vi "Check if Notifier is Registered.vi"(8 "error in (no error)":errorcluster, 11 "name (unnamed)":string) -> (0 "error out":errorcluster, 1 "Registered?":bool, 3 "Registered Notifier":refnum<notifier>)   [LabVIEW 2023]
doc: "This VI checks to see if a queue is in the Queue Registry.\n\nIf the queue is in the registry, Registered? is true and the queue is returned. If it is not, Registred is false and an empty queue is returned."
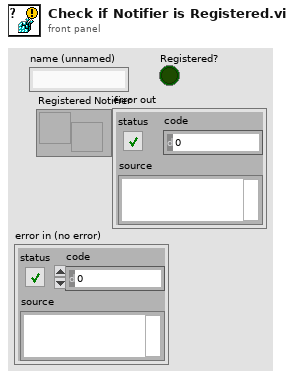
[diagram p1: front panel]
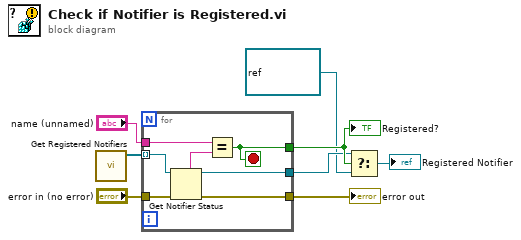
[diagram p0: block diagram]
diagram:
  n1 = call "Get Registered Notifiers.vi"() -> ("Notifier References"=w2:refnum<notifier>[])  [unwired: 10 in, 1 out]
  n2 = for {
    tunnel: w2 -> [w13] mode=indexing
    tunnel: "name (unnamed)" -> [w15]
    tunnel: [w10] -> w4
    tunnel: [w14] -> w5
    tunnel: "error in (no error)" -> [w12]
    tunnel: [w9] -> w6
    stop <- w14 stop-if-true
    n3 = Get Notifier Status(notifier=w13, error in (no error)=w12) -> (notifier out=w10:refnum<notifier>, notifier name=w11:string, error out=w9:errorcluster)  [unwired: 2 out]
    n4 = Equal?(x=w15, y=w11) -> (x = y?=w14:bool)
  }
  "Registered?" <- w5
  "error out" <- w6
  n5 = Select(t=w4, s=w5, f=refnum<notifier> refnum ("notifier out")) -> (s? t:f=→"Registered Notifier":refnum<notifier>)
